vi "main_init_reactor_tipstrip.vi"(10 "Reactor legend":refnum<vi>) -> ()   [LabVIEW 2019]
uses:
  <vilib>/picture/picture.llb/imagedata.ctl
panel:
  out "feedback pic":T1
  out "storage pic":T1
  out "hydrolysis pic":T1
  out "methane pic":T1
  # "*******************************************************************\nBiogas Plant Control\n\nAuthor: Paul Zügel\nGCSC-Frankfurt am Main 2020\n\n*******************************************************************"
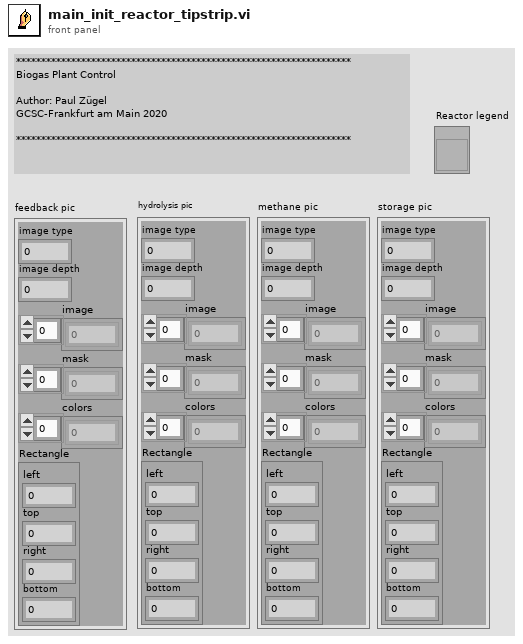
[diagram p1: front panel]
types:
  T1 = typedef "imagedata.ctl" = cluster{"image type":i32, "image depth":i32, "image":u8[], "mask":u8[], "colors":u32[], "Rectangle":cluster{"left":i16, "top":i16, "right":i16, "bottom":i16}}
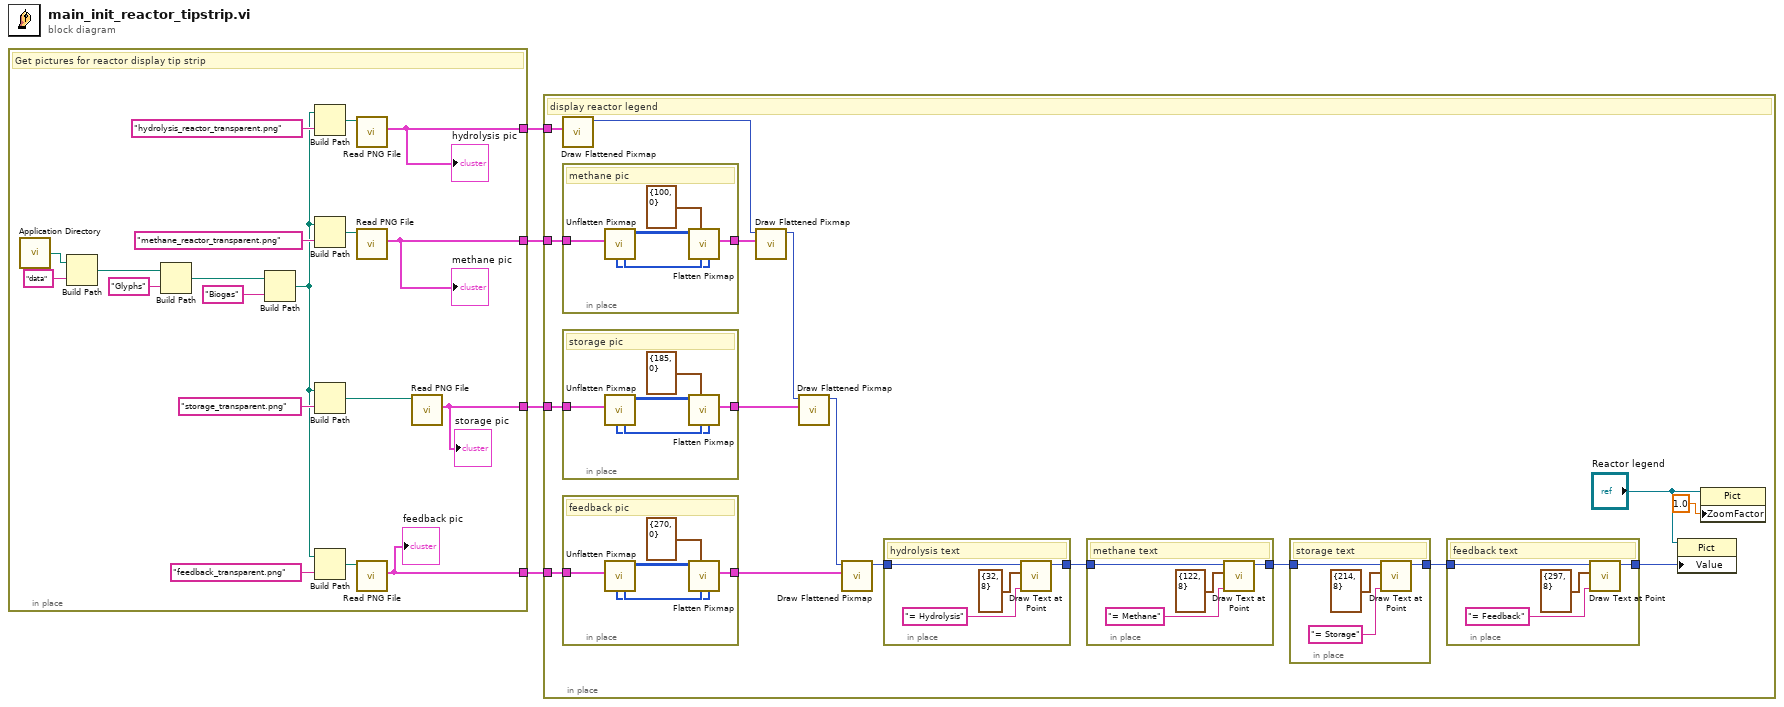
[diagram p0: block diagram]
diagram:
  n1 = in-place {
    in-place-border: [w8] -> w4
    in-place-border: [w7] -> w3
    in-place-border: [w6] -> w2
    in-place-border: [w5] -> w1
    # "Get pictures for reactor display tip strip"
    n2 = call <vilib>:"Application Directory.vi"() -> ("Application Directory"=w23:path)
    n3 = Build Path(base path=w23, name or relative path="data") -> (appended path=w21:path)
    n4 = Build Path(base path=w21, name or relative path="Glyphs") -> (appended path=w19:path)
    n5 = Build Path(base path=w19, name or relative path="Biogas") -> (appended path=w9:path)
    n6 = Build Path(base path=w9, name or relative path="hydrolysis_reactor_transparent.png") -> (appended path=w16:path)
    n7 = Build Path(base path=w9, name or relative path="methane_reactor_transparent.png") -> (appended path=w14:path)
    n8 = Build Path(base path=w9, name or relative path="storage_transparent.png") -> (appended path=w12:path)
    n9 = Build Path(base path=w9, name or relative path="feedback_transparent.png") -> (appended path=w10:path)
    n10 = call <vilib>:"Read PNG File.vi"("path to PNG file"=w16) -> ("image data"=w5:T1)  [unwired: 8 in, 2 out]
    "hydrolysis pic" <- w5
    n11 = call <vilib>:"Read PNG File.vi"("path to PNG file"=w14) -> ("image data"=w8:T1)  [unwired: 8 in, 2 out]
    "methane pic" <- w8
    n12 = call <vilib>:"Read PNG File.vi"("path to PNG file"=w10) -> ("image data"=w6:T1)  [unwired: 8 in, 2 out]
    "feedback pic" <- w6
    n13 = call <vilib>:"Read PNG File.vi"("path to PNG file"=w12) -> ("image data"=w7:T1)  [unwired: 8 in, 2 out]
    "storage pic" <- w7
  }
  n14 = in-place {
    in-place-border: w4 -> [w27]
    in-place-border: w3 -> [w26]
    in-place-border: w2 -> [w25]
    in-place-border: w1 -> [w24]
    # "display reactor legend"
    n15 = call <vilib>:"Draw Flattened Pixmap.vi"("image data"=w24) -> ("new picture"=w39:picture)  [unwired: 8 in]
    n16 = in-place {
      in-place-border: [w59] -> w40
      in-place-border: w27 -> [w57]
      # "methane pic"
      n17 = call <vilib>:"Unflatten Pixmap.vi"("image data"=w57) -> ("24-bit pixmap"=w62:u32[][], "colors"=w61:u32[], "mask"=w60:u8[])  [unwired: 4 in, 4 out]
      n18 = call <vilib>:"Flatten Pixmap.vi"("mask"=w60, "colors"=w61, "top left"=cluster{"x":i16, "y":i16} {"x"=100, "y"=0}, "24-bit pixmap"=w62) -> ("image data"=w59:T1)  [unwired: 7 in]
    }
    n19 = in-place {
      in-place-border: [w52] -> w36
      in-place-border: w26 -> [w51]
      # "storage pic"
      n20 = call <vilib>:"Unflatten Pixmap.vi"("image data"=w51) -> ("24-bit pixmap"=w56:u32[][], "colors"=w55:u32[], "mask"=w54:u8[])  [unwired: 4 in, 4 out]
      n21 = call <vilib>:"Flatten Pixmap.vi"("mask"=w54, "colors"=w55, "top left"=cluster{"x":i16, "y":i16} {"x"=185, "y"=0}, "24-bit pixmap"=w56) -> ("image data"=w52:T1)  [unwired: 7 in]
    }
    n22 = in-place {
      in-place-border: [w46] -> w32
      in-place-border: w25 -> [w45]
      # "feedback pic"
      n23 = call <vilib>:"Unflatten Pixmap.vi"("image data"=w45) -> ("24-bit pixmap"=w50:u32[][], "colors"=w49:u32[], "mask"=w48:u8[])  [unwired: 4 in, 4 out]
      n24 = call <vilib>:"Flatten Pixmap.vi"("mask"=w48, "colors"=w49, "top left"=cluster{"x":i16, "y":i16} {"x"=270, "y"=0}, "24-bit pixmap"=w50) -> ("image data"=w46:T1)  [unwired: 7 in]
    }
    n25 = call <vilib>:"Draw Flattened Pixmap.vi"("image data"=w40, "picture"=w39) -> ("new picture"=w37:picture)  [unwired: 7 in]
    n26 = call <vilib>:"Draw Flattened Pixmap.vi"("image data"=w36, "picture"=w37) -> ("new picture"=w31:picture)  [unwired: 7 in]
    n27 = call <vilib>:"Draw Flattened Pixmap.vi"("image data"=w32, "picture"=w31) -> ("new picture"=w30:picture)  [unwired: 7 in]
    n28 = in-place {
      in-place-border: [w64] -> w38
      in-place-border: w30 -> [w63]
      # "hydrolysis text"
      n29 = call <vilib>:"Draw Text at Point.vi"("text"="= Hydrolysis", "origin"=cluster{"x":i16, "y":i16} {"x"=32, "y"=8}, "picture"=w63) -> ("new picture"=w64:picture)  [unwired: 7 in, 1 out]
    }
    n30 = in-place {
      in-place-border: w38 -> [w70]
      in-place-border: [w67] -> w35
      # "methane text"
      n31 = call <vilib>:"Draw Text at Point.vi"("text"="= Methane", "origin"=cluster{"x":i16, "y":i16} {"x"=122, "y"=8}, "picture"=w70) -> ("new picture"=w67:picture)  [unwired: 7 in, 1 out]
    }
    n32 = in-place {
      in-place-border: w35 -> [w74]
      in-place-border: [w73] -> w29
      # "storage text"
      n33 = call <vilib>:"Draw Text at Point.vi"("text"="= Storage", "origin"=cluster{"x":i16, "y":i16} {"x"=214, "y"=8}, "picture"=w74) -> ("new picture"=w73:picture)  [unwired: 7 in, 1 out]
    }
    n34 = in-place {
      in-place-border: [w44] -> w28
      in-place-border: w29 -> [w41]
      # "feedback text"
      n35 = call <vilib>:"Draw Text at Point.vi"("text"="= Feedback", "origin"=cluster{"x":i16, "y":i16} {"x"=297, "y"=8}, "picture"=w41) -> ("new picture"=w44:picture)  [unwired: 7 in, 1 out]
    }
    n36 = property on="Property Node" class="Pict"(reference="Reactor legend", "Value"=w28) -> ()  [unwired: 1 in, 2 out]
    n37 = property class="Pict"(reference="Reactor legend", "ZoomFactor"=sgl 1.0 ("Zoom Factor")) -> ()  [unwired: 1 in, 2 out]
  }
